vi "test_lin_int_FFT.vi"() -> ()   [LabVIEW 2009]
doc: "Copyright (C) 2009, Stepan A. Baranov\nweb: http://www.OCTLab.org/\nemail: stepan@baranov.su"
uses:
  <vilib>/Analysis/4window.llb/Hanning Window (DBL).vi
  <vilib>/Analysis/NI_AALPro.lvlib
  OCTLib.dll
  <vilib>/gmath/NI_Gmath.lvlib
panel:
  out "error out":errorcluster
  out "Im part":dbl[](array[numeric])
  out "Re part":dbl[](array[numeric])
  out "Phase A-scan":dbl[](array[numeric])
  out "Intensity A-scan":dbl[](array[numeric])
  out "Im":dbl[](array[numeric])
  out "Re":dbl[](array[numeric])
  out "phase":dbl[](array[numeric])
  out "intensity":dbl[](array[numeric])
  out "time for FFT":u32
  in  "RSM_STAT?":bool=TRUE
  in  "stop":bool
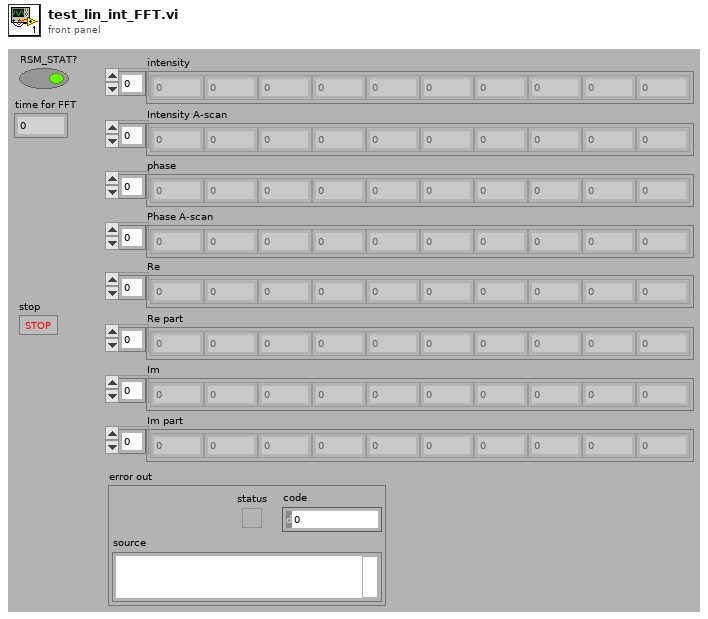
[diagram p1: front panel]
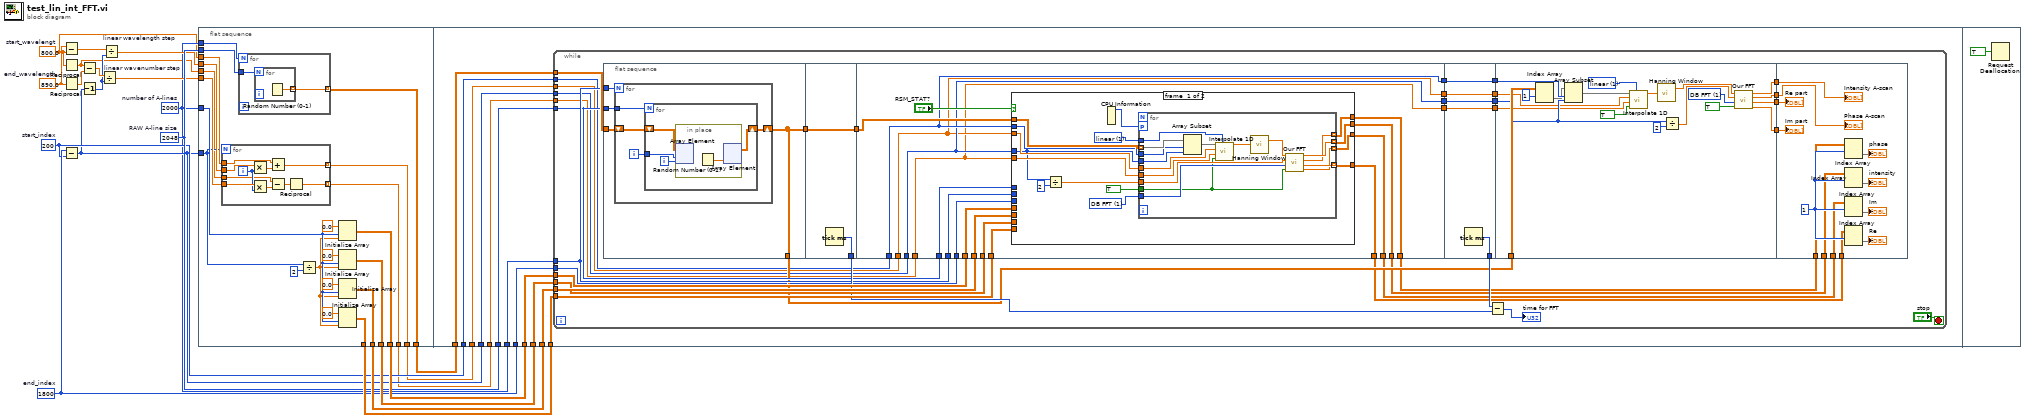
[diagram p0: block diagram]
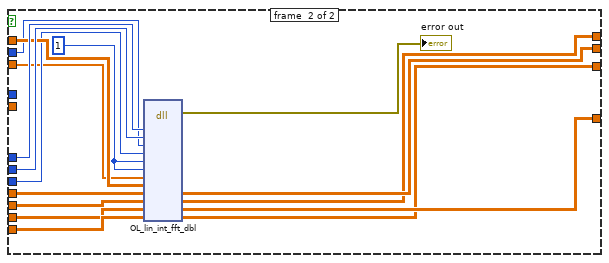
[diagram p2: hidden frame]
diagram:
  w1 = 800.0  # start_wavelengt
  w9 = 890.0  # end_wavelength
  w15 = 1800  # end_index
  w8 = 200  # start_index
  w4 = 2000  # number of A-lines
  w16 = 2048  # RAW A-line size
  n1 = Subtract(x=w9, y=w1) -> (x-y=w14:dbl)
  n2 = Reciprocal(x=w1) -> (1/x=w2:dbl)
  n3 = Reciprocal(x=w9) -> (1/x=w3:dbl)
  n4 = Subtract(x=w15, y=w8) -> (x-y=w7:i32)
  n5 = Subtract(x=w2, y=w3) -> (x-y=w13:dbl)
  n6 = Decrement(x=w7) -> (x-1=w12:i32)
  n7 = Divide "linear wavenumber step"(x=w13, y=w12) -> (x/y=w11:dbl)
  n8 = Divide "linear wavelength step"(x=w14, y=w12) -> (x/y=w10:dbl)
  n9 = flat-sequence {
    tunnel: w16 -> [w42]
    tunnel: w4 -> [w41]
    tunnel: w4 -> [w36]
    tunnel: [w35] -> w21
    tunnel: [w34] -> w20
    tunnel: [w33] -> w19
    tunnel: [w32] -> w18
    tunnel: [w31] -> w17
    tunnel: w7 -> [w26]
    tunnel: w11 -> [w30]
    tunnel: w10 -> [w29]
    tunnel: w1 -> [w28]
    tunnel: [w22] -> w6
    tunnel: [w27] -> w5
    tunnel: w2 -> [w23]
    tunnel: w4 -> [w67]
    tunnel: w16 -> [w66]
    tunnel: w21 -> [w65]
    tunnel: w20 -> [w64]
    tunnel: w19 -> [w63]
    tunnel: w18 -> [w62]
    tunnel: w17 -> [w61]
    tunnel: w8 -> [w60]
    tunnel: w15 -> [w59]
    tunnel: w7 -> [w58]
    tunnel: w6 -> [w57]
    tunnel: w5 -> [w56]
    frame #0 {
      n10 = for {
        N: w26 -> [_]
        tunnel: w30 -> [w52]
        tunnel: [w44] -> w27 mode=indexing
        tunnel: w29 -> [w49]
        tunnel: w28 -> [w48]
        tunnel: [w43] -> w22 mode=indexing
        tunnel: w23 -> [w46]
        i -> [w50]
        n11 = Multiply(x=w49, y=w50) -> (x*y=w47:dbl)
        n12 = Multiply(x=w52, y=w50) -> (x*y=w51:dbl)
        n13 = Add(x=w48, y=w47) -> (x+y=w43:dbl)
        n14 = Subtract(x=w46, y=w51) -> (x-y=w45:dbl)
        n15 = Reciprocal(x=w45) -> (1/x=w44:dbl)
      }
      n16 = for {
        N: w41 -> [_]
        tunnel: [w54] -> w31 mode=indexing
        tunnel: w42 -> [w53]
        n17 = for {
          N: w53 -> [_]
          tunnel: [w55] -> w54 mode=indexing
          n18 = Random Number (0-1)() -> (number: 0 to 1=w55:dbl)
        }
      }
      n19 = Divide(x=w26, y=2) -> (x/y=w24:dbl)
      n20 = Initialize Array(0.0 ("element"), w36, w24) -> (w34:dbl[][])
      n21 = Initialize Array(0.0 ("element"), w36, w24) -> (w33:dbl[][])
      n22 = Initialize Array(0.0 ("element"), w36, w24) -> (w35:dbl[][])
      n23 = Initialize Array(0.0 ("element"), w36, w24) -> (w32:dbl[][])
    }
    frame #1 {
      n24 = while {
        tunnel: w61 -> [w101]
        tunnel: w67 -> [w93]
        tunnel: w66 -> [w92]
        tunnel: w65 -> [w100]
        tunnel: w64 -> [w99]
        tunnel: w63 -> [w98]
        tunnel: w62 -> [w97]
        tunnel: w60 -> [w80]
        tunnel: w59 -> [w79]
        tunnel: w58 -> [w78]
        tunnel: w57 -> [w77]
        tunnel: w56 -> [w76]
        stop <- "stop" stop-if-true
        n25 = flat-sequence {
          tunnel: w101 -> [w106]
          tunnel: w93 -> [w105]
          tunnel: w92 -> [w104]
          tunnel: [w103] -> w91
          tunnel: [w103] -> w81
          tunnel: [w117] -> w96
          tunnel: [w116] -> w82
          tunnel: w81 -> [w116]
          tunnel: w100 -> [w133]
          tunnel: w99 -> [w132]
          tunnel: w98 -> [w131]
          tunnel: w97 -> [w130]
          tunnel: w92 -> [w129]
          tunnel: w93 -> [w128]
          tunnel: [w127] -> w86
          tunnel: [w126] -> w85
          tunnel: [w125] -> w84
          tunnel: [w124] -> w83
          tunnel: w82 -> [w123]
          tunnel: w80 -> [w121]
          tunnel: w79 -> [w122]
          tunnel: w78 -> [w120]
          tunnel: w77 -> [w119]
          tunnel: w76 -> [w118]
          tunnel: [w121] -> w74
          tunnel: [w120] -> w72
          tunnel: [w119] -> w71
          tunnel: [w118] -> w68
          tunnel: [w186] -> w94
          tunnel: [w185] -> w75
          tunnel: w74 -> [w185]
          tunnel: [w184] -> w73
          tunnel: w72 -> [w184]
          tunnel: w71 -> [w183]
          tunnel: [w183] -> w70
          tunnel: [w182] -> w69
          tunnel: w68 -> [w182]
          tunnel: w91 -> [w206]
          tunnel: [w201] -> w90
          tunnel: [w200] -> w89
          tunnel: [w199] -> w88
          tunnel: [w198] -> w87
          tunnel: w75 -> [w197]
          tunnel: w73 -> [w196]
          tunnel: w70 -> [w190]
          tunnel: w69 -> [w189]
          tunnel: w90 -> [w219]
          tunnel: w89 -> [w218]
          tunnel: w88 -> [w217]
          tunnel: w87 -> [w216]
          tunnel: w86 -> [w214]
          tunnel: w85 -> [w212]
          tunnel: w84 -> [w210]
          tunnel: w83 -> [w208]
          frame #0 {
            n26 = for {
              N: w105 -> [_]
              shift-right: [w108] -> w103
              shift-left: w106 -> [w109]
              tunnel: w104 -> [w110]
              i -> [w107]
              n27 = for {
                N: w110 -> [_]
                shift-right: [w111] -> w108
                shift-left: w109 -> [w114]
                tunnel: w107 -> [w113]
                i -> [w112]
                n28 = in-place {
                  n29 = in-place-array #1(w114, w113, w112) -> ()  [unwired: 1 out]
                  n30 = Random Number (0-1)() -> (number: 0 to 1=w115:dbl)
                  n31 = in-place-array #1(w115) -> (w111:dbl[][])  [unwired: 2 out]
                }
              }
            }
          }
          frame #1 {
            n32 = Tick Count (ms)() -> (millisecond timer value=w117:u32)
          }
          frame #2 {
            n33 = case shown="True" "RSM_STAT?" {
              tunnel: w133 -> [_ w178]
              tunnel: w132 -> [_ w181]
              tunnel: w131 -> [_ w180]
              tunnel: w130 -> [_ w179]
              tunnel: w129 -> [_ w177]
              tunnel: w128 -> [_ w176]
              tunnel: w123 -> [w149 w174]
              tunnel: [w145 w173] -> w127
              tunnel: [w144 w172] -> w126
              tunnel: [w143 w171] -> w125
              tunnel: [w142 w170] -> w124
              tunnel: w121 -> [w141 w169]
              tunnel: w122 -> [_ w168]
              tunnel: w120 -> [w138 _]
              tunnel: w119 -> [w140 w166]
              tunnel: w118 -> [w139 _]
              frame #0 {
                w135 = 1 items=["nearest", "linear", "spline", "cubic Hermite", "Lagrange"] ("method")
                w146 = 1 items=["LINEAR FFT", "DB FFT"] ("A-scan type")
                n34 = Divide(x=w138, y=2) -> (x/y=w136:dbl)
                n35 = CPU Information() -> (4:w148:i32)  [unwired: 3 out]
                n36 = for {
                  workers-P: w148 -> [_]
                  tunnel: [w164] -> w145 mode=indexing
                  tunnel: [w163] -> w144 mode=indexing
                  tunnel: [w162] -> w143 mode=indexing
                  tunnel: [w161] -> w142 mode=indexing
                  tunnel: w149 -> [w159] mode=indexing
                  tunnel: TRUE ("need phase?") -> [w151]
                  tunnel: w146 -> [w160]
                  tunnel: w141 -> [w158]
                  tunnel: w138 -> [w157]
                  tunnel: w140 -> [w154]
                  tunnel: w139 -> [w153]
                  tunnel: w136 -> [w156]
                  tunnel: w135 -> [w150]
                  n37 = Array Subset(array=w159, index=w158, length=w157) -> (w155:dbl[])
                  n38 = call <vilib>:"Interpolate 1D.vi"("method"=w150, "X is monotonic"=w151, "xi"=w153, "X"=w154, "Y"=w155) -> ("yi"=w152:dbl[])  [unwired: 4 in, 2 out]
                  n39 = call-poly <vilib>:"Hanning Window.vi"("X"=w152) -> ("Windowed X"=w165:dbl[])  [unwired: 1 out]
                  n40 = call "Our FFT.vi"("need phase?"=w151, "A-scan type"=w160, "FFT A-scan size"=w156, "RAW A-line"=w165) -> ("Im part"=w161:dbl[], "Re part"=w162:dbl[], "Phase A-scan"=w163:dbl[], "Intensity A-scan"=w164:dbl[])
                }
              }
              frame #1 {
                w175 = i8 1 ("hanning_flag")
                n41 = dll-call lib="OCTLib.dll" fn="OL_lin_int_fft_dbl"("width"=w177, "height"=w176, "start_index"=w169, "end_index"=w168, "hanning_flag"=w175, "log10_flag"=w175, "spectrum"=w166, "input"=w174, "intensity"=w181, "phase"=w180, "Re"=w178, "Im"=w179) -> (error out=→"error out":errorcluster, "intensity"=w173:dbl[][], "phase"=w172:dbl[][], "Re"=w171:dbl[][], "Im"=w170:dbl[][])  [unwired: 12 in, 1 out]
              }
            }
          }
          frame #3 {
            n42 = Tick Count (ms)() -> (millisecond timer value=w186:u32)
          }
          frame #4 {
            w192 = 1 items=["nearest", "linear", "spline", "cubic Hermite", "Lagrange"] ("method")
            w203 = 1 items=["LINEAR FFT", "DB FFT"] ("A-scan type")
            n43 = Index Array(array=w206, index (row)=1) -> (element=w191:dbl[])  [unwired: 1 in]
            n44 = Array Subset(array=w191, index=w197, length=w196) -> (w187:dbl[])
            n45 = call <vilib>:"Interpolate 1D.vi"("method"=w192, "X is monotonic"=TRUE, "xi"=w189, "X"=w190, "Y"=w187) -> ("yi"=w188:dbl[])  [unwired: 4 in, 2 out]
            n46 = call-poly <vilib>:"Hanning Window.vi"("X"=w188) -> ("Windowed X"=w204:dbl[])  [unwired: 1 out]
            n47 = Divide(x=w196, y=2) -> (x/y=w194:dbl)
            n48 = call "Our FFT.vi"("need phase?"=TRUE, "A-scan type"=w203, "FFT A-scan size"=w194, "RAW A-line"=w204) -> ("Im part"=w198:dbl[], "Re part"=w199:dbl[], "Phase A-scan"=w200:dbl[], "Intensity A-scan"=w201:dbl[])
          }
          frame #5 {
            w215 = 1 ("index (row)")
            n49 = Index Array(array=w212, index (row)=w215) -> (element=→"phase":dbl[])  [unwired: 1 in]
            n50 = Index Array(array=w214, index (row)=w215) -> (element=→"intensity":dbl[])  [unwired: 1 in]
            n51 = Index Array(array=w208, index (row)=w215) -> (element=→"Im":dbl[])  [unwired: 1 in]
            n52 = Index Array(array=w210, index (row)=w215) -> (element=→"Re":dbl[])  [unwired: 1 in]
            "Intensity A-scan" <- w219
            "Phase A-scan" <- w218
            "Re part" <- w217
            "Im part" <- w216
          }
        }
        n53 = Subtract(x=w94, y=w96) -> (x-y=→"time for FFT":u32)
      }
    }
    frame #2 {
      n54 = Request Deallocation(TRUE ("flag")) -> ()
    }
  }
